vi "Translate_TABPAGES.vi"(8 "error IN":errorcluster, 10 "Cle":string, 11 "TabCtl Refnum":refnum<vi>) -> (0 "error out":errorcluster)   [LabVIEW 2013]
uses:
  Dictionnary/EnumCommandDictionnaire.ctl
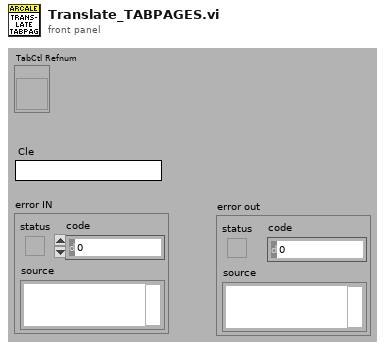
[diagram p1: front panel]
types:
  T1 = typedef "EnumCommandDictionnaire.ctl" = enum16{"Load", "Translate", "Save", "GetDico", "Set : A traduire = Vrai", "Set : A Traduire = Faux", "SetDico"}
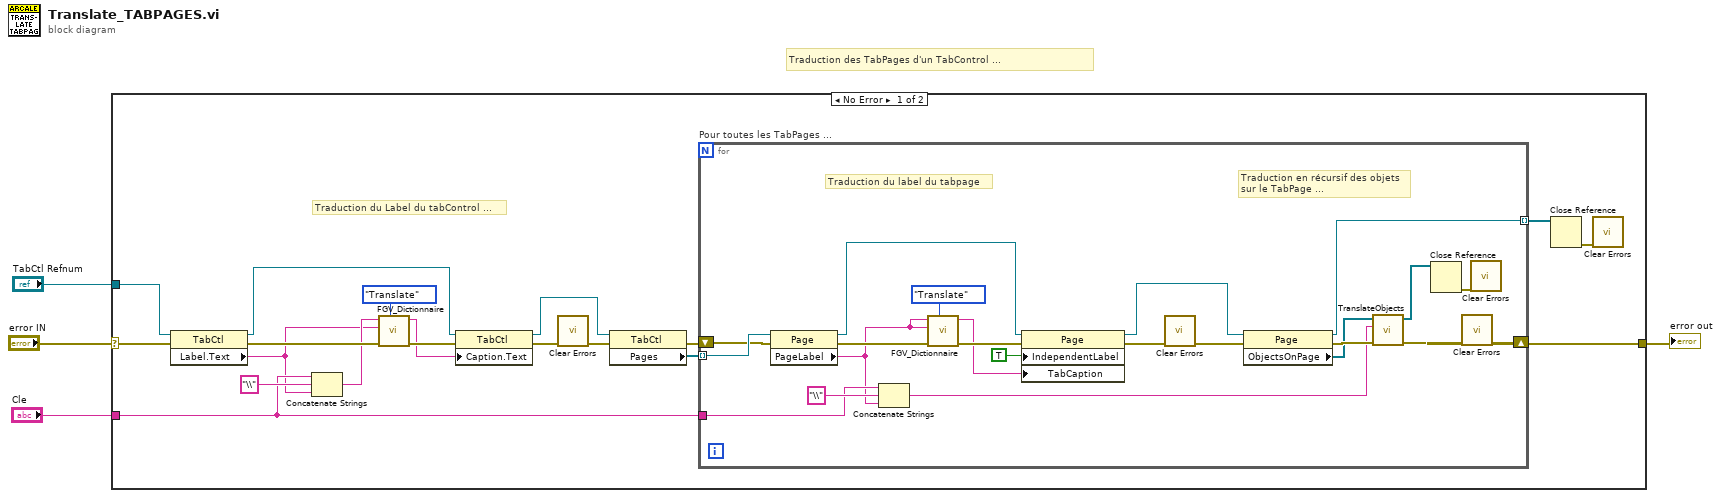
[diagram p0: block diagram]
diagram:
  # "Traduction des TabPages d'un TabControl ..."
  n1 = case shown="No Error" "error IN" {
    selector: "error IN" -> [w18 w46]
    tunnel: "TabCtl Refnum" -> [w17 _]
    tunnel: "Cle" -> [w13 _]
    tunnel: [w21 w46] -> w1
    frame No Error {
      # "Traduction du Label du tabControl ..."
      n2 = property class="TabCtl"(reference=w17, error in=w18) -> (reference out=w7:refnum<vi>, error out=w15:errorcluster, "Label.Text"=w11:string)
      n3 = Concatenate Strings(w13, "\\" ("string"), w11) -> (w12:string)
      n4 = call "FGV_Dictionnaire.vi"("Command"=EnumCommandDictionnaire."Translate", "error in (no error)"=w15, "Chaîne"=w11, "Clé"=w12) -> ("error out"=w10:errorcluster, "Traduction"=w8:string)  [unwired: 5 in, 1 out]
      n5 = property class="TabCtl"(reference=w7, error in=w10, "Caption.Text"=w8) -> (reference out=w5:refnum<vi>, error out=w9:errorcluster)
      n6 = call <vilib>:"Clear Errors.vi"("error in (no error)"=w9) -> ("error out"=w6:errorcluster)  [unwired: 6 in]
      n7 = property class="TabCtl"(reference=w5, error in=w6) -> (error out=w22:errorcluster, "Pages"=w23:refnum<vi>[])  [unwired: 1 out]
      n8 = for "Pour toutes les TabPages ..." {
        tunnel: w23 -> [w45] mode=indexing
        tunnel: w13 -> [w35]
        shift-right: [w28] -> w21
        shift-left: w22 -> [w44]
        tunnel: [w26] -> w20 mode=indexing
        # "Traduction en récursif des objets\nsur le TabPage ..."
        # "Traduction du label du tabpage"
        n9 = property class="Page"(reference=w45, error in=w44) -> (reference out=w27:refnum<vi>, error out=w33:errorcluster, "PageLabel"=w24:string)
        n10 = Concatenate Strings(w35, "\\" ("string"), w24) -> (w29:string)
        n11 = call "FGV_Dictionnaire.vi"("Command"=EnumCommandDictionnaire."Translate", "error in (no error)"=w33, "Chaîne"=w24, "Clé"=w24) -> ("error out"=w32:errorcluster, "Traduction"=w31:string)  [unwired: 5 in, 1 out]
        n12 = property class="Page"(reference=w27, error in=w32, "IndependentLabel"=TRUE ("Independent Label"), "TabCaption"=w31) -> (reference out=w41:refnum<vi>, error out=w42:errorcluster)
        n13 = call <vilib>:"Clear Errors.vi"("error in (no error)"=w42) -> ("error out"=w25:errorcluster)  [unwired: 6 in]
        n14 = property class="Page"(reference=w41, error in=w25) -> (reference out=w26:refnum<vi>, error out=w40:errorcluster, "ObjectsOnPage"=w39:refnum<vi>[])
        n15 = call "TranslateObjects.vi"("errorIN"=w40, "Cle"=w29, "AllObjs[]In"=w39) -> ("error out"=w38:errorcluster, "AllObjs[]Out"=w37:refnum<vi>[])  [unwired: 7 in]
        n16 = Close Reference(reference=w37) -> (error out=w36:errorcluster)  [unwired: 1 in]
        n17 = call <vilib>:"Clear Errors.vi"("error in (no error)"=w38) -> ("error out"=w28:errorcluster)  [unwired: 6 in]
        n18 = call <vilib>:"Clear Errors.vi"("error in (no error)"=w36) -> ()  [unwired: 6 in, 1 out]
      }
      n19 = Close Reference(reference=w20) -> (error out=w19:errorcluster)  [unwired: 1 in]
      n20 = call <vilib>:"Clear Errors.vi"("error in (no error)"=w19) -> ()  [unwired: 6 in, 1 out]
    }
    frame Error {
    }
  }
  "error out" <- w1
